vi "ParseArguments.vi"(6 "arguments name":string="args", 7 "parser name":string="parser", 8 "error in":errorcluster, 11 "VI Interpreter in":refnum<class "VI Interpreter.lvclass">) -> (0 "error out":errorcluster, 3 "VI Interpreter out":refnum<class "VI Interpreter.lvclass">, 5 "python assignment":string)   [LabVIEW 2014, in "PyConvBD.lvclass"]
uses:
  PyConvBD.lvclass
  VI Interpreter/Classes/VI Interpreter/VI Interpreter.lvclass
  Parsing/Python Functions.lvlib
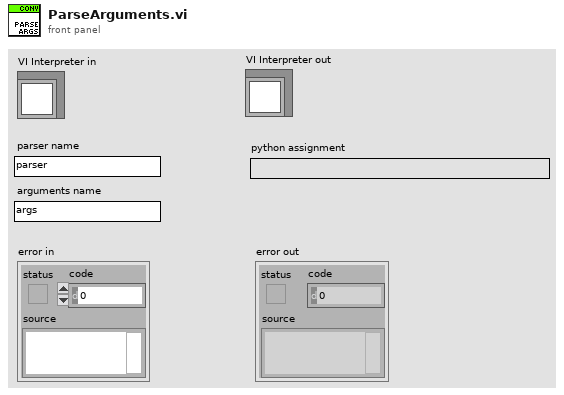
[diagram p1: front panel]
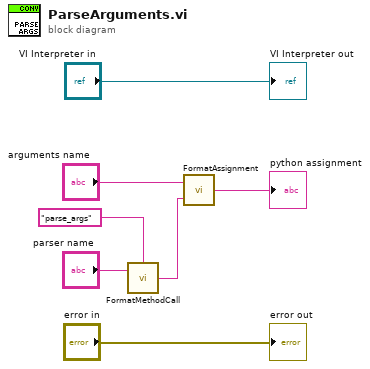
[diagram p0: block diagram]
diagram:
  n1 = call "FormatMethodCall.vi"("method"="parse_args", "object"="parser name") -> ("python object"=w3:string)  [unwired: 1 in]
  n2 = call "FormatAssignment.vi"("value"=w3, "name"="arguments name") -> ("python assignment"=→"python assignment":string)
  "error out" <- "error in"
  "VI Interpreter out" <- "VI Interpreter in"
